vi "1_SimpleDemo_MHHisto.vi"() -> ()   [LabVIEW 2017]
uses:
  _lib/PQ/MultiHarp/MH_RefSource.ctl
  _lib/PQ/MultiHarp/MH_MeasMode.ctl
  <vilib>/Utility/error.llb/Error Cluster From Error Code.vi
  _lib/PQ/MultiHarp/MH_LibVersion_global.vi
  _lib/PQ/MultiHarp/mhlib_x86_x64_UIThread.llb/MH_DllPath_global.vi
  <vilib>/ErrorRing/Error Ring.xnode
panel:
  in  "EnableInputDeadTime":bool caption="Enable DeadTime"
  in  "InputDeadTime":i32=1000 caption="DeadTime [ps]" min=800 max=160000 step=1
  in  "Trg.Edge":i32(ring) items=["falling", "rising"]
  in  "Trg.Level":i32=-100 caption="Trg.Level [mV]" min=-1200 max=1200 step=1
  in  "Offset":i32 caption="Offset [ps]" min=-99999 max=99999 step=1
  in  "Enable":bool=TRUE
  in  "EnableSyncDeadTime":bool caption="Enable DeadTime"
  in  "SyncDeadTime":i32=1000 caption="SyncDeadTime [ps]" min=800 max=160000 step=1
  in  "SyncTrg.Edge":i32(ring) items=["falling", "rising"]
  in  "SyncTrg.Level":i32=-100 caption="SyncTrg.Level [mV]" min=-1200 max=1200 step=1
  in  "SyncOffset":i32 caption="SyncOffset [ps]" min=-99999 max=99999 step=1
  in  "SyncDivider":i32(ring)=1 items=["1"=1, "2"=2, "4"=4, "8"=8, "16"=16]
  in  "Binning":i32(ring) caption="Resolution [ps]" items=["10 / 80", "20 / 160", "40 / 320", "80 / 640", "160 / 1280", "320 / 2560", "640 / 5120", "1280 / 10240", "2560 / 20480", "5120 / 40960", "10240 / 81920", "20480 / 163840", "40960 / 327680", "81920 / 655360", "163840 / 1310720", "327680 / 2621440", "655360 / 5242880", "1310720 / 10485760", "2621440 / 20971520", "5242880 / 41943040", "10485760 / 83886080", "20971520 / 167772160", "41943040 / 335544320"]
  in  "HistoLength":i32(ring)=6 caption="Histo Length" items=["1024", "2048", "4096", "8192", "16384", "32768", "65536"]
  in  "Acqu.Time":i32=10000 caption="Acqu.Time [ms]" min=1 max=360000 step=1
  in  "GlobalOffset":i32 caption="GlobalOffset [ns]" min=0 max=100000000 step=1
  in  "OverflowLevel":u32=4294967295 min=1 step=1
  in  "StopOnOverflow":bool=TRUE
  out "HistoGraph":T1(graph)={0.0, "Resolution"=0.08, "Histogram"=array8x65536[524288 elements]}
  out "CountRates":i32[](array[numeric]) caption="Count Rates [cps]"
  out "SyncRate":i32 caption="Sync Rate [cps]"
  in  "stop":bool
  out "error out":errorcluster
  # "All Channels"
  # "Sync"
  # "Acquisition"
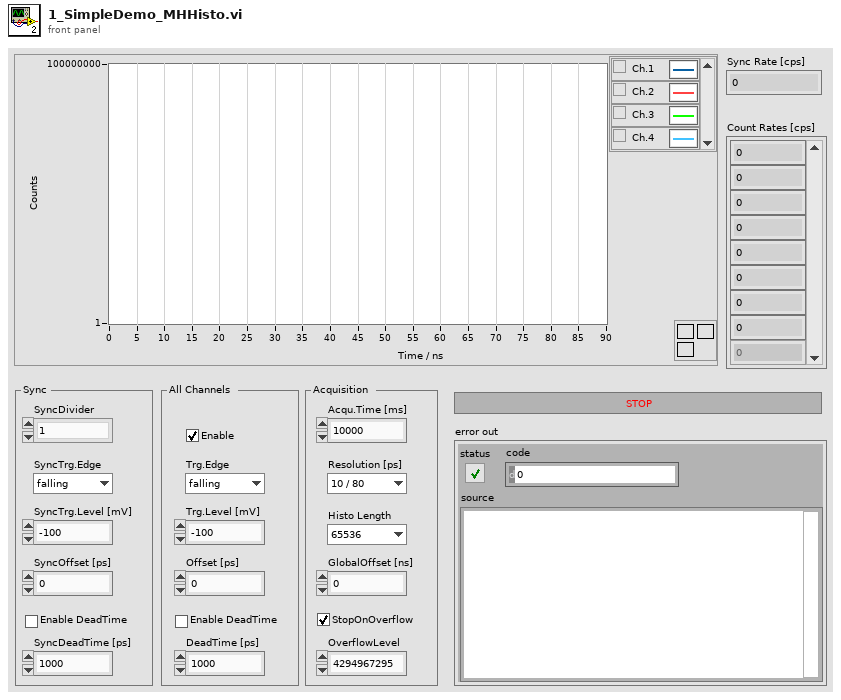
[diagram p1: front panel]
types:
  T1 = cluster{dbl, "Resolution":dbl, "Histogram":u32[][]}
  T2 = typedef "MH_MeasMode.ctl" = i32
  T3 = typedef "MH_RefSource.ctl" = enum16{"INTERNAL", "EXTERNAL_10MHZ", "WR_MASTER_GENERIC", "WR_SLAVE_GENERIC", "WR_GRANDM_GENERIC", "EXTN_GPS_PPS", "EXTN_GPS_PPS_UART", "WR_MASTER_MHARP", "WR_SLAVE_MHARP", "WR_GRANDM_MHARP"}
  T4 = typedef "MH_InitInfo.ctl" = cluster{"Library Version":string, "Serial No.":string, "Model":string, "Partnum":string, "Version":string, "features":i32, "nchannels":i32, "Base Resolution":dbl, "Bin Steps":i32}
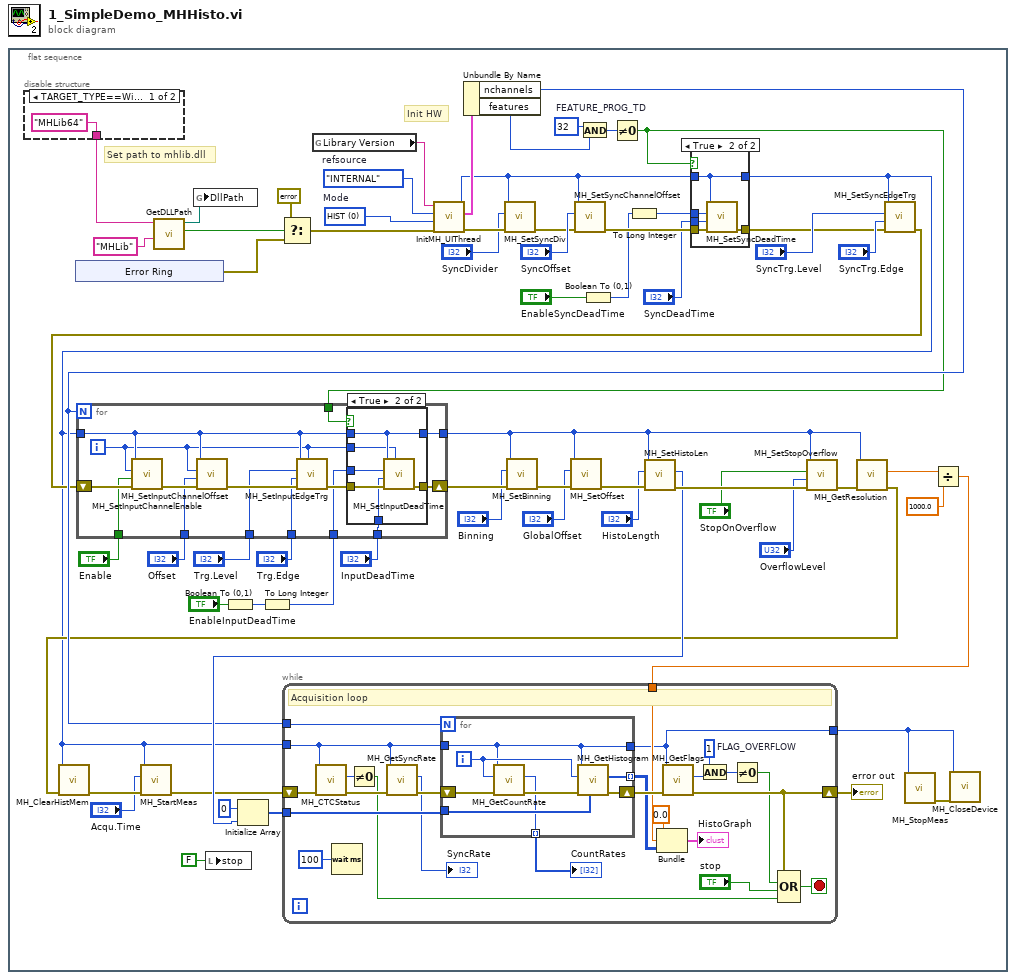
[diagram p0: block diagram]
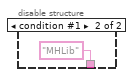
[diagram p3: hidden frame]
diagram:
  n1 = flat-sequence {
    frame #0 {
      w7 = 32  # FEATURE_PROG_TD
      w18 = T2 0 items=["HIST"=0, "T2"=2, "T3"=3]  # Mode
      w64 = MH_RefSource."INTERNAL"  # refsource
      # "Init HW"
      # "Set path to mhlib.dll"
      n2 = disable-structure shown="TARGET_TYPE==Windows, Default" {
        disable-tunnel: ["MHLib64" ("name or relative path") "MHLib" ("name or relative path")] -> w17
        frame condition #0 (active) {
        }
        frame condition #1 {
        }
      }
      n3 = xnode "Error Ring"() -> ("error out"=w63:errorcluster)
      n4 = call "GetDLLPath.vi"("DllName_32bit"="MHLib" ("name or relative path"), "DllName_64bit"=w17) -> ("file exists?"=w61:bool, "DLLPath"=w60:path)  [unwired: 8 in]
      n5 = global write "MH_DllPath_global.vi" "DllPath"(w60) -> ()
      n6 = local write "stop"(FALSE ("stop")) -> ()
      n7 = Boolean To (0,1)(Boolean="EnableInputDeadTime") -> (0, 1=w3:i16)
      n8 = To Long Integer(number=w3) -> (32bit integer=w2:i32)
      n9 = Select(t=errorcluster {"status"=FALSE, "code"=0, "source"=""} ("error IO"), s=w61, f=w63) -> (s? t:f=w58:errorcluster)
      n10 = global read "MH_LibVersion_global.vi" "Library Version"() -> (w21:string)
      n11 = call "InitMH_UIThread.vi"("error in (no error)"=w58, "Mode"=w18, "refsource"=w64, "Library Version"=w21) -> ("error out"=w53:errorcluster, "Init Info"=w55:T4, "DevIdx"=w14:i32)  [unwired: 5 in]
      n12 = Unbundle By Name(w55) -> ("nchannels"=w35:i32, "features"=w9:i32)
      n13 = call "MH_SetSyncDiv.vi"("error in (no error)"=w53, "SyncDivider"="SyncDivider", "devidx"=w14) -> ("error out"=w52:errorcluster)  [unwired: 7 in, 1 out]
      n14 = call "MH_SetSyncChannelOffset.vi"("error in (no error)"=w52, "Offset"="SyncOffset", "devidx"=w14) -> ("error out"=w16:errorcluster)  [unwired: 7 in, 1 out]
      n15 = And(x=w7, y=w9) -> (x .and. y?=w8:i32)
      n16 = Boolean To (0,1)(Boolean="EnableSyncDeadTime") -> (0, 1=w12:i16)
      n17 = Not Equal To 0?(x=w8) -> (x != 0?=w1:bool)
      n18 = To Long Integer(number=w12) -> (32bit integer=w11:i32)
      n19 = case shown="True" w1 {
        tunnel: w16 -> [w65 w71]
        tunnel: [w65 w70] -> w15
        tunnel: w14 -> [w66 w67]
        tunnel: w11 -> [_ w69]
        tunnel: "SyncDeadTime" -> [_ w68]
        tunnel: [w66 w67] -> w6
        frame False {
        }
        frame True {
          n20 = call "MH_SetSyncDeadTime.vi"("error in (no error)"=w71, "deadtime"=w68, "on"=w69, "devidx"=w67) -> ("error out"=w70:errorcluster)  [unwired: 6 in, 1 out]
        }
      }
      n21 = call "MH_SetSyncEdgeTrg.vi"("error in (no error)"=w15, "edge"="SyncTrg.Edge", "level"="SyncTrg.Level", "devidx"=w6) -> ("error out"=w34:errorcluster)  [unwired: 6 in, 1 out]
      n22 = for {
        N: w35 -> [_]
        shift-right: [w111] -> w54
        shift-left: w34 -> [w120]
        tunnel: w6 -> [w112]
        tunnel: [w110] -> w29
        tunnel: "Enable" -> [w117]
        tunnel: "Offset" -> [w116]
        tunnel: "Trg.Edge" -> [w115]
        tunnel: "Trg.Level" -> [w114]
        tunnel: "InputDeadTime" -> [w108]
        tunnel: w2 -> [w107]
        tunnel: w1 -> [w106]
        i -> [w109]
        n23 = call "MH_SetInputChannelEnable.vi"("error in (no error)"=w120, "enable"=w117, "channel"=w109, "devidx"=w112) -> ("error out"=w119:errorcluster)  [unwired: 6 in, 1 out]
        n24 = call "MH_SetInputChannelOffset.vi"("error in (no error)"=w119, "Offset"=w116, "channel"=w109, "devidx"=w112) -> ("error out"=w118:errorcluster)  [unwired: 6 in, 1 out]
        n25 = call "MH_SetInputEdgeTrg.vi"("channel"=w109, "error in (no error)"=w118, "edge"=w115, "level"=w114, "devidx"=w112) -> ("error out"=w113:errorcluster)  [unwired: 5 in, 1 out]
        n26 = case shown="True" w106 {
          tunnel: w113 -> [w122 w128]
          tunnel: w112 -> [w121 w126]
          tunnel: [w122 w127] -> w111
          tunnel: [w121 w126] -> w110
          tunnel: w109 -> [_ w125]
          tunnel: w108 -> [_ w124]
          tunnel: w107 -> [_ w123]
          frame False {
          }
          frame True {
            n27 = call "MH_SetInputDeadTime.vi"("channel"=w125, "error in (no error)"=w128, "deadtime"=w124, "on"=w123, "devidx"=w126) -> ("error out"=w127:errorcluster)  [unwired: 5 in, 1 out]
          }
        }
      }
      n28 = call "MH_SetBinning.vi"("error in (no error)"=w54, "Binning"="Binning", "devidx"=w29) -> ("error out"=w50:errorcluster)  [unwired: 7 in, 1 out]
      n29 = call "MH_SetOffset.vi"("error in (no error)"=w50, "Offset"="GlobalOffset", "devidx"=w29) -> ("error out"=w48:errorcluster)  [unwired: 7 in, 1 out]
      n30 = call "MH_SetHistoLen.vi"("error in (no error)"=w48, "lencode"="HistoLength", "devidx"=w29) -> ("error out"=w47:errorcluster, "actuallen"=w40:i32)  [unwired: 6 in, 1 out]
      n31 = Initialize Array(u32 0, w40) -> (w39:u32[])
      n32 = call "MH_SetStopOverflow.vi"("error in (no error)"=w47, "stopcount"="OverflowLevel", "StopOnOverflow"="StopOnOverflow", "devidx"=w29) -> ("error out"=w30:errorcluster)  [unwired: 6 in, 1 out]
      n33 = call "MH_GetResolution.vi"("error in (no error)"=w30, "devidx"=w29) -> ("error out"=w27:errorcluster, "resolution"=w28:dbl)  [unwired: 7 in, 1 out]
      n34 = call "MH_ClearHistMem.vi"("error in (no error)"=w27, "devidx"=w6) -> ("error out"=w44:errorcluster)  [unwired: 8 in, 1 out]
      n35 = call "MH_StartMeas.vi"("error in (no error)"=w44, "tacq"="Acqu.Time", "devidx"=w6) -> ("error out"=w26:errorcluster)  [unwired: 7 in, 1 out]
      n36 = Divide(x=w28, y=1000.0) -> (x/y=w36:dbl)
      n37 = while {
        shift-right: [w85] -> w42
        shift-left: w26 -> [w96]
        tunnel: w6 -> [w92]
        tunnel: w35 -> [w95]
        tunnel: w39 -> [w87]
        tunnel: w36 -> [w79]
        tunnel: [w74] -> w20
        stop <- w86 stop-if-true
        w90 = 1  # FLAG_OVERFLOW
        # "Acquisition loop"
        n38 = call "MH_CTCStatus.vi"("error in (no error)"=w96, "devidx"=w92) -> ("error out"=w94:errorcluster, "ctcstatus"=w97:i32)  [unwired: 7 in, 1 out]
        n39 = Wait (ms)(milliseconds to wait=u32 100) -> ()  [unwired: 1 out]
        n40 = Not Equal To 0?(x=w97) -> (x != 0?=w76:bool)
        n41 = call "MH_GetSyncRate.vi"("error in (no error)"=w94, "devidx"=w92) -> ("error out"=w93:errorcluster, "syncrate"=→"SyncRate":i32)  [unwired: 7 in, 1 out]
        n42 = for {
          N: w95 -> [_]
          shift-right: [w105] -> w91
          shift-left: w93 -> [w104]
          tunnel: w92 -> [w101]
          tunnel: [w101] -> w74
          tunnel: w87 -> [w100]
          tunnel: [w99] -> w82 mode=indexing
          tunnel: [w98] -> w81 mode=indexing
          i -> [w102]
          n43 = call "MH_GetCountRate.vi"("error in (no error)"=w104, "Channel"=w102, "devidx"=w101) -> ("error out"=w103:errorcluster, "rate"=w99:i32)  [unwired: 6 in, 1 out]
          n44 = call "MH_GetHistogram.vi"("Chcount"=w100, "error in (no error)"=w103, "channel"=w102, "devidx"=w101) -> ("error out"=w105:errorcluster, "Histogram"=w98:u32[])  [unwired: 5 in, 1 out]
        }
        "CountRates" <- w82
        n45 = Bundle(0.0, w79, "Histogram"=w81) -> (→"HistoGraph":cluster{dbl, dbl, "Histogram":u32[][]})  [unwired: 1 in]
        n46 = call "MH_GetFlags.vi"("error in (no error)"=w91, "devidx"=w74) -> ("error out"=w85:errorcluster, "flags"=w88:i32)  [unwired: 7 in, 1 out]
        n47 = And(x=w90, y=w88) -> (x .and. y?=w89:i32)
        n48 = Not Equal To 0?(x=w89) -> (x != 0?=w84:bool)
        n49 = Compound Arithmetic op=OR(w85, w84, "stop", w76) -> (w86:bool)
      }
      "error out" <- w42
      n50 = call "MH_StopMeas.vi"("devidx"=w20) -> ("error out"=w19:errorcluster)  [unwired: 9 in, 1 out]
      n51 = call "MH_CloseDevice.vi"("error in (no error)"=w19, "devidx"=w20) -> ()  [unwired: 8 in, 2 out]
    }
  }
